vi "Graph1D2D.vi"(0 "#pts2":u32=2, 3 "DataSel":u16(ring) items=["D0", "D1", "D2", "D3"], 4 "#pts1":u32=21, 5 "Data":dbl[][](array[numeric]), 6 "Axis2":dbl[](array[numeric]), 7 "Axis1":dbl[](array[numeric])) -> (1 "2Dplot":dbl[][](graph), 2 "1Dplot":cluster{"Axis1":dbl[], dbl[]}[](graph))   [LabVIEW 2022 SP3]
panel:
  out "appended array":dbl[](array[numeric])
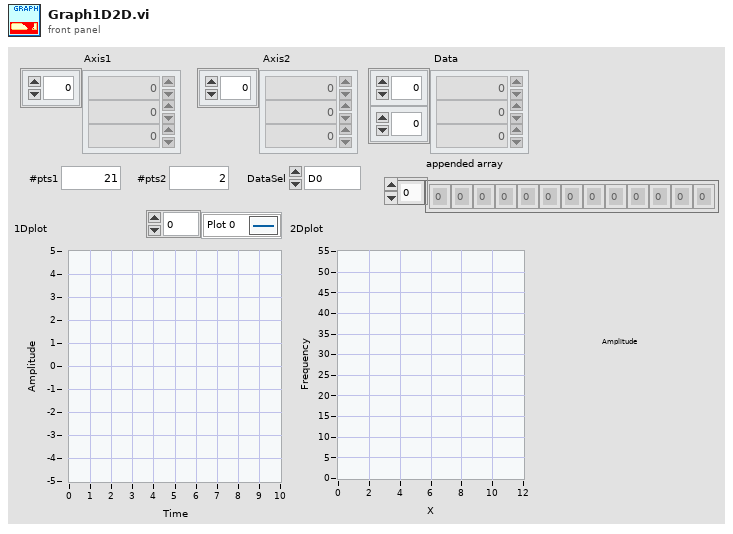
[diagram p1: front panel]
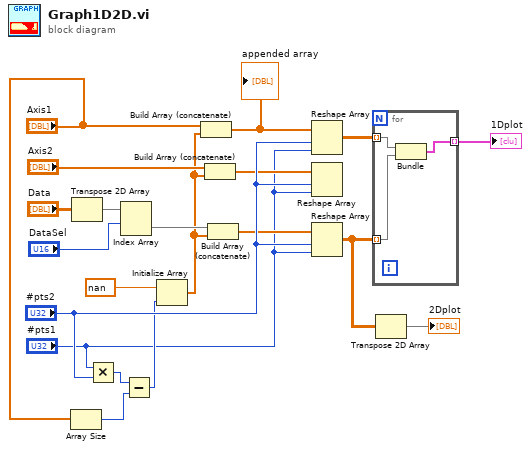
[diagram p0: block diagram]
diagram:
  n1 = Array Size(array="Axis1") -> (size(s)=w13:i32)
  n2 = Transpose 2D Array(2D array="Data") -> (transposed array=w19:dbl[][])
  n3 = Multiply(x="#pts1", y="#pts2") -> (x*y=w14:u32)
  n4 = Index Array(array=w19, index (row)="DataSel") -> (element=w8:dbl[])  [unwired: 1 in]
  n5 = Subtract(x=w14, y=w13) -> (x-y=w12:u32)
  n6 = Initialize Array(nan, w12) -> (w5:dbl[])
  n7 = Build Array (concatenate)("Axis1", w5) -> (w9:dbl[])
  "appended array" <- w9
  n8 = Build Array (concatenate)("Axis2", w5) -> (w4:dbl[])
  n9 = Build Array (concatenate)(w8, w5) -> (w7:dbl[])
  n10 = Reshape Array(w9, "#pts2", "#pts1") -> (w17:dbl[][])
  n11 = Reshape Array(w4, "#pts2", "#pts1") -> ()  [unwired: 1 out]
  n12 = Reshape Array(w7, "#pts2", "#pts1") -> (w2:dbl[][])
  n13 = for {
    tunnel: w17 -> [w23] mode=indexing
    tunnel: w2 -> [w22] mode=indexing
    tunnel: [w21] -> w16 mode=indexing
    n14 = Bundle(w23, w22) -> (w21:cluster{dbl[], dbl[]})  [unwired: 1 in]
  }
  "1Dplot" <- w16
  n15 = Transpose 2D Array(2D array=w2) -> (transposed array=→"2Dplot":dbl[][])
